vi "Default Quad Channels.vi"(1 "Channels":T3={"# Input Channels"=0, "# Output Channels"=0, "Channel Type"=enum."Digital", "Units"=""}) -> (0 "Quadrature":T1 {"Quadrature Channels"."Index Mode" items=["Disabled", "Phase B0 A0", "Phase B0 A1", "Phase B1 A0", "Phase B1 A1"]; "Quadrature Channels"."Timebase" items=["256 us", "512 us", "1024 us", "2048 us", "4096 us", "8192 us", "16384 us", "32768 us"]})   [LabVIEW 2011, in "Modules.lvlib" / "SD Module.lvclass"]
uses:
  SD Module.lvclass
  RSI Module/Channels.ctl
  RSI Module/Channel Type.ctl
  Type Defs/Quadrature.ctl
  Type Defs/Quadrature Channel.ctl
  RSI Module/RSI Module.lvclass
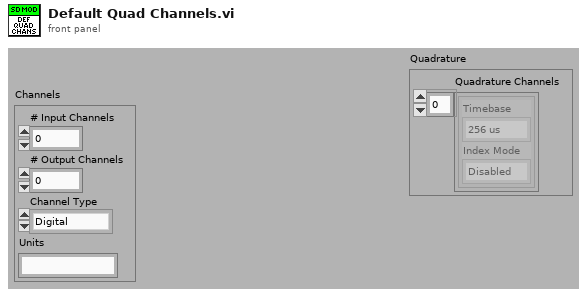
[diagram p1: front panel]
types:
  T1 = typedef "Modules.lvlib/SD Module.lvclass/Quadrature.ctl" = cluster{"Quadrature Channels":T2[]}
  T2 = typedef "Modules.lvlib/SD Module.lvclass/Quadrature Channel.ctl" = cluster{"Timebase":u32, "Index Mode":u32}
  T3 = typedef "Modules.lvlib/RSI Module.lvclass/Channels.ctl" = cluster{"# Input Channels":i32, "# Output Channels":i32, "Channel Type":T4, "Units":string}
  T4 = typedef "Modules.lvlib/RSI Module.lvclass/Channel Type.ctl" = enum16{"Analog", "Digital"}
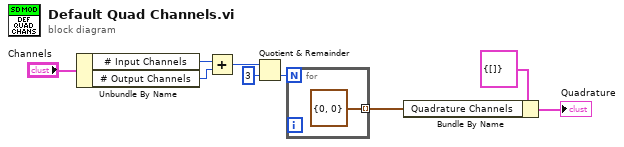
[diagram p0: block diagram]
diagram:
  n1 = Unbundle By Name("Channels") -> ("# Input Channels"=w3:i32, "# Output Channels"=w2:i32)
  n2 = Add(x=w3, y=w2) -> (x+y=w1:i32)
  n3 = Quotient & Remainder(x=w1, y=3) -> (floor(x/y)=w4:i32)  [unwired: 1 out]
  n4 = for {
    N: w4 -> [_]
    tunnel: [T2 {"Timebase"=0, "Index Mode"=0} ("Quadrature Channel")] -> w9 mode=indexing
  }
  n5 = Bundle By Name(cluster=T1 {"Quadrature Channels"=[]} ("Quadrature"), "Quadrature Channels"=w9) -> (→"Quadrature":T1)
